vi "Join myDAQ DIO.vi"(5 "IN 7":bool, 6 "IN 5":bool, 7 "IN 6, IN 4":fxp<+,2,2> format="%02b", 8 "IN 2, IN 0":fxp<+,2,2> format="%02b", 9 "IN 3":bool, 10 "IN 1":bool) -> (2 "IN 7:0":u8 format="%08b")   [LabVIEW 2014]
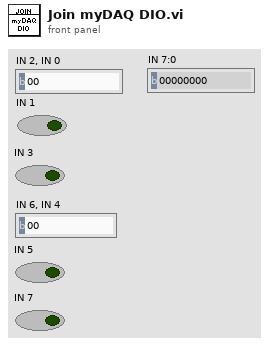
[diagram p1: front panel]
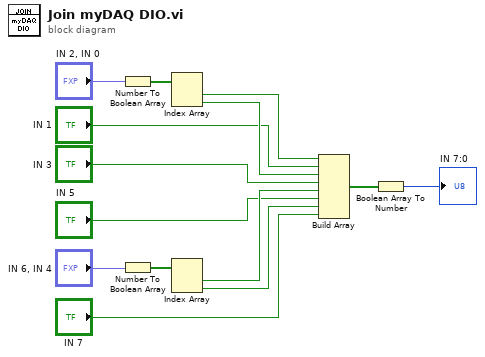
[diagram p0: block diagram]
diagram:
  n1 = Number To Boolean Array(number="IN 2, IN 0") -> (Boolean array=w14:bool[])
  n2 = Number To Boolean Array(number="IN 6, IN 4") -> (Boolean array=w13:bool[])
  n3 = Index Array(array=w14) -> (element #1=w10:bool, element #2=w9:bool)  [unwired: 2 in]
  n4 = Index Array(array=w13) -> (element #1=w6:bool, element #2=w5:bool)  [unwired: 2 in]
  n5 = Build Array(w10, "IN 1", w9, "IN 3", w6, "IN 5", w5, "IN 7") -> (w2:bool[])
  n6 = Boolean Array To Number(Boolean array=w2) -> (number=→"IN 7:0":u8)
